vi "rt nominal disconnect.vi"(8 "error in":errorcluster, 11 "nominal state":T1) -> (0 "error out":errorcluster)   [LabVIEW 2026, in "Nominal Core Streaming Engine.lvlib"]
uses:
  Nominal Core Streaming Engine.lvlib
  nominal runtime state.ctl
  Shared/time convert type.ctl
  lib_nominal-streaming-lv_64.dll
  Shared/Nominal Core Streaming Shared.lvlib
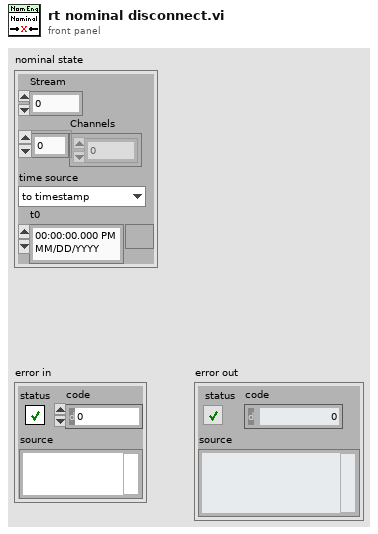
[diagram p1: front panel]
types:
  T1 = typedef "Nominal Core Streaming Engine.lvlib/nominal runtime state.ctl" = cluster{"Stream":u64, "Channels":u64[], "time source":T2, "t0":timestamp}
  T2 = typedef "Nominal Core Streaming Shared.lvlib/time convert type.ctl" = enum16{"to timestamp", "relative seconds"}
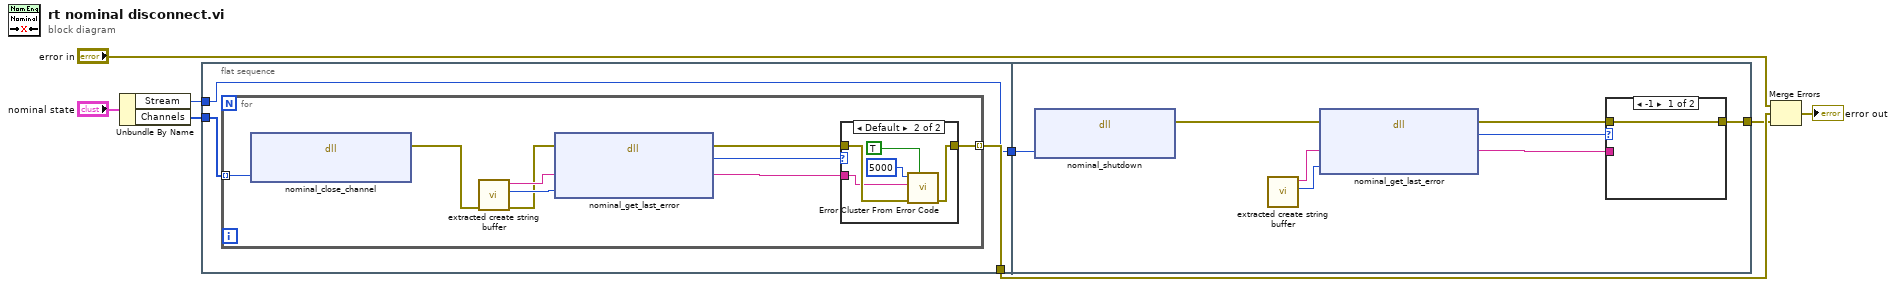
[diagram p0: block diagram]
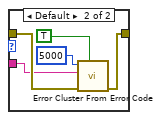
[diagram p3: hidden frame]
diagram:
  n1 = Unbundle By Name("nominal state") -> ("Stream"=w2:u64, "Channels"=w7:u64[])
  n2 = flat-sequence {
    tunnel: w7 -> [w11]
    tunnel: [w10] -> w5
    tunnel: w2 -> [w9]
    tunnel: [w9] -> w1
    tunnel: [w33] -> w4
    tunnel: w1 -> [w34]
    frame #0 {
      n3 = for {
        tunnel: w11 -> [w20] mode=indexing
        tunnel: [w19] -> w10 mode=indexing
        n4 = dll-call lib="C:/sw/ni-veristand-custom-device-nominal-core/source/lib_nominal-streaming-lv_*.*" fn="nominal_close_channel"("writer_handle"=w20) -> (error out=w13:errorcluster)  [unwired: 5 in, 1 out]
        n5 = call "extracted create string buffer.vi"("error in"=w13) -> ("error out"=w12:errorcluster, "dub Buffer Size"=w14:i32, "String Buffer"=w15:string)  [unwired: 8 in]
        n6 = dll-call lib="C:/sw/ni-veristand-custom-device-nominal-core/source/lib_nominal-streaming-lv_*.*" fn="nominal_get_last_error"(error in=w12, "buffer"=w15, "buffer_size"=w14) -> (error out=w16:errorcluster, "return type"=w18:i32, "buffer"=w17:string)  [unwired: 3 in, 1 out]
        n7 = case shown="Default" w18 {
          tunnel: w16 -> [w21 w26]
          tunnel: [w21 w25] -> w19
          tunnel: w17 -> [_ w24]
          frame -1 {
          }
          frame Default {
            n8 = call <vilib>:"Error Cluster From Error Code.vi"("show call chain? (False)"=TRUE, "error in (no error)"=w26, "error message (\"\")"=w24, "error code (0)"=5000) -> ("error out"=w25:errorcluster)  [unwired: 5 in]
          }
        }
      }
    }
    frame #1 {
      n9 = dll-call lib="C:/sw/ni-veristand-custom-device-nominal-core/source/lib_nominal-streaming-lv_*.*" fn="nominal_shutdown"("stream_handle"=w34) -> (error out=w32:errorcluster)  [unwired: 5 in, 1 out]
      n10 = call "extracted create string buffer.vi"() -> ("dub Buffer Size"=w27:i32, "String Buffer"=w28:string)  [unwired: 9 in, 1 out]
      n11 = dll-call lib="C:/sw/ni-veristand-custom-device-nominal-core/source/lib_nominal-streaming-lv_*.*" fn="nominal_get_last_error"(error in=w32, "buffer"=w28, "buffer_size"=w27) -> (error out=w29:errorcluster, "return type"=w31:i32, "buffer"=w30:string)  [unwired: 3 in, 1 out]
      n12 = case shown="-1" w31 {
        tunnel: w29 -> [w35 w40]
        tunnel: [w35 w39] -> w33
        tunnel: w30 -> [_ w38]
        frame -1 {
        }
        frame Default {
          n13 = call <vilib>:"Error Cluster From Error Code.vi"("show call chain? (False)"=TRUE, "error in (no error)"=w40, "error message (\"\")"=w38, "error code (0)"=5000) -> ("error out"=w39:errorcluster)  [unwired: 5 in]
        }
      }
    }
  }
  n14 = Merge Errors("error in", w5, w4) -> (→"error out":errorcluster)
